vi "GetContent.vi"(8 "Error In":errorcluster, 11 "reference in":refnum<class "Text.lvclass">) -> (0 "Error Out":errorcluster, 2 "Content":string, 3 "reference out":refnum<class "Text.lvclass">)   [LabVIEW 2024, in "Text.lvclass"]
uses:
  Text.lvclass
  Text.lvclass/Text.ctl
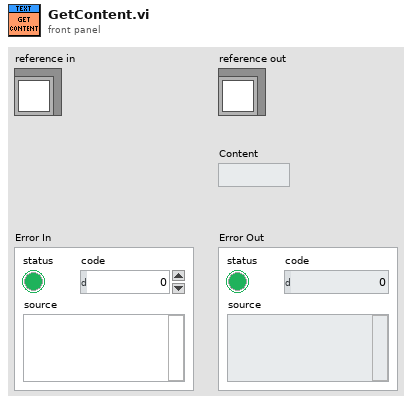
[diagram p1: front panel]
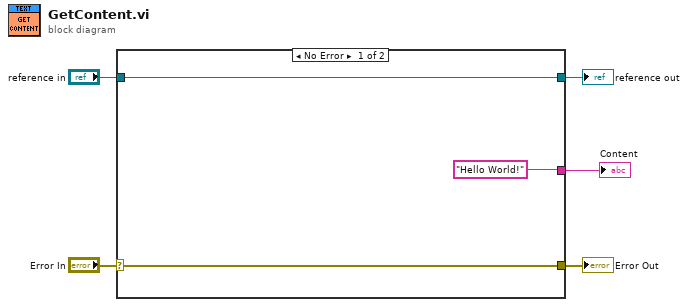
[diagram p0: block diagram]
diagram:
  n1 = case shown="No Error" "Error In" {
    selector: "Error In" -> [w7 w10]
    tunnel: [w7 w10] -> w4
    tunnel: [w8 w9] -> w2
    tunnel: "reference in" -> [w8 w9]
    tunnel: ["Hello World!" _] -> w1
    frame No Error {
    }
    frame Error {
    }
  }
  "Error Out" <- w4
  "reference out" <- w2
  "Content" <- w1
